vi "GetSubList.vi"(8 "error in (no error)":errorcluster, 9 "ParentTag(Empty for Top)":string, 11 "CMenu in":refnum<class "CMenu.lvclass">) -> (0 "error out":errorcluster, 1 "SubList":T1(array[cluster]), 3 "CMenu out":refnum<class "CMenu.lvclass">)   [LabVIEW 2020, in "CMenu.lvclass"]
uses:
  CMenu.lvclass
  CMenu.lvclass/CMenu.ctl
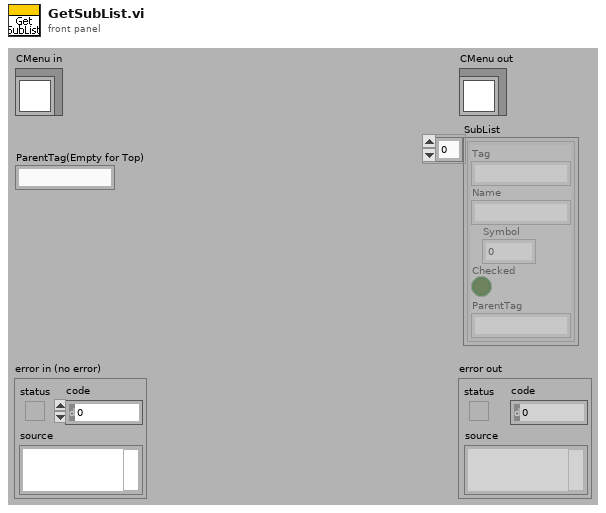
[diagram p1: front panel]
types:
  T1 = cluster{"Tag":string, "Name":string, "Symbol":i32, "Checked":bool, "ParentTag":string}[]
  T2 = cluster{"Tag":string, "Caption":string, "Symbol":i32, "Checked":bool, "ParentTag":string}[]
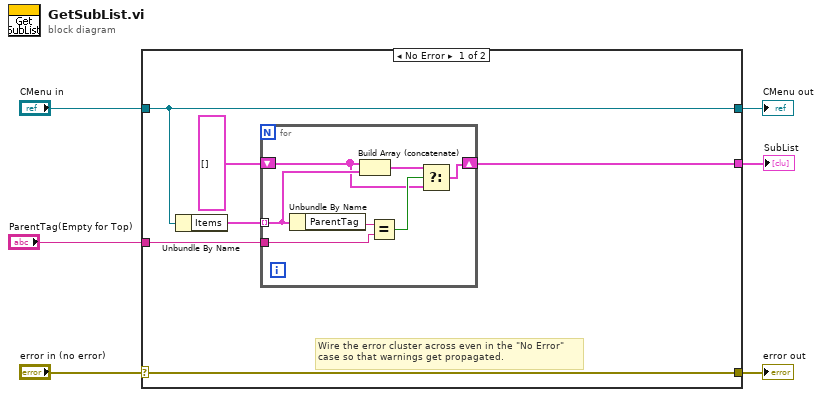
[diagram p0: block diagram]
diagram:
  n1 = case shown="No Error" "error in (no error)" {
    selector: "error in (no error)" -> [w12 w21]
    tunnel: [w12 w21] -> w5
    tunnel: [w11 w20] -> w3
    tunnel: "CMenu in" -> [w11 w20]
    tunnel: [w8 _] -> w2
    tunnel: "ParentTag(Empty for Top)" -> [w7 _]
    frame No Error {
      # "Wire the error cluster across even in the \"No Error\"\ncase so that warnings get propagated."
      n2 = Unbundle By Name(w11) -> ("Items"=w10:T1)
      n3 = for {
        tunnel: w10 -> [w18] mode=indexing
        shift-right: [w14] -> w8
        shift-left: T2 [] -> [w16]
        tunnel: w7 -> [w13]
        n4 = Unbundle By Name(w18) -> ("ParentTag"=w19:string)
        n5 = Build Array (concatenate)(w16, w18) -> (w15:T1)
        n6 = Equal?(x=w19, y=w13) -> (x = y?=w17:bool)
        n7 = Select(t=w15, s=w17, f=w16) -> (s? t:f=w14:T2)
      }
    }
    frame Error {
    }
  }
  "error out" <- w5
  "CMenu out" <- w3
  "SubList" <- w2
